vi "MFCI_RESPONSE.vi"(0 "Input":string) -> (1 "Match?":bool, 2 "Channel":i32, 3 "Data":dbl)   [LabVIEW 2011]
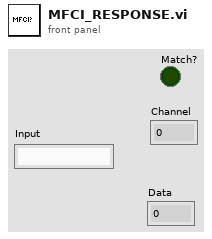
[diagram p1: front panel]
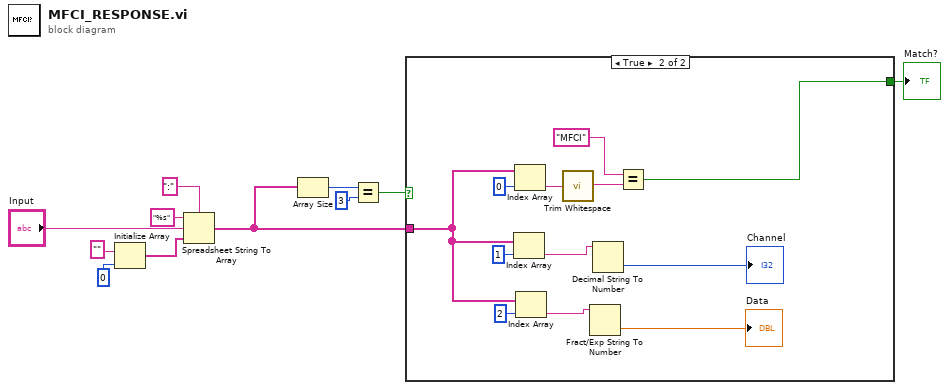
[diagram p0: block diagram]
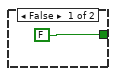
[diagram p2: hidden frame]
diagram:
  n1 = Initialize Array("", 0) -> (w9:string[])
  n2 = Spreadsheet String To Array(delimiter (Tab)=":", format string="%s", spreadsheet string="Input", array type (2D Dbl)=w9) -> (array=w2:string[])
  n3 = Array Size(array=w2) -> (size(s)=w5:i32)
  n4 = Equal?(x=w5, y=3) -> (x = y?=w3:bool)
  n5 = case shown="True" w3 {
    tunnel: w2 -> [_ w24]
    tunnel: [FALSE w13] -> w1
    frame False {
    }
    frame True {
      n6 = Index Array(array=w24, index=1) -> (element=w17:string)
      n7 = Index Array(array=w24, index=0) -> (element=w20:string)
      n8 = Index Array(array=w24, index=2) -> (element=w15:string)
      n9 = call <vilib>:"Trim Whitespace.vi"("string"=w20) -> ("trimmed string"=w19:string)  [unwired: 1 in]
      n10 = Fract/Exp String To Number(string=w15) -> (number=→"Data":dbl)  [unwired: 3 in, 1 out]
      n11 = Decimal String To Number(string=w17) -> (number=→"Channel":i32)  [unwired: 2 in, 1 out]
      n12 = Equal?(x="MFCI", y=w19) -> (x = y?=w13:bool)
    }
  }
  "Match?" <- w1
